vi "SplineFit.vi"(10 "Y array":dbl[](array[numeric]), 11 "X array":dbl[](array[numeric])) -> (2 "derivative":cluster{dbl[], "Best Polynomial Fit":dbl[]}[](graph), 3 "Spline":cluster{dbl[], "dX/dt":dbl[]}(graph), 4 "w_r":dbl, 5 "Point":cluster{dbl[], dbl[]})   [LabVIEW 2022 SP3]
uses:
  <vilib>/gmath/NI_Gmath.lvlib
  <vilib>/Analysis/NI_AALPro.lvlib
panel:
  out "error":i32
  out "Polynomial Coefficients":dbl[](array[numeric])
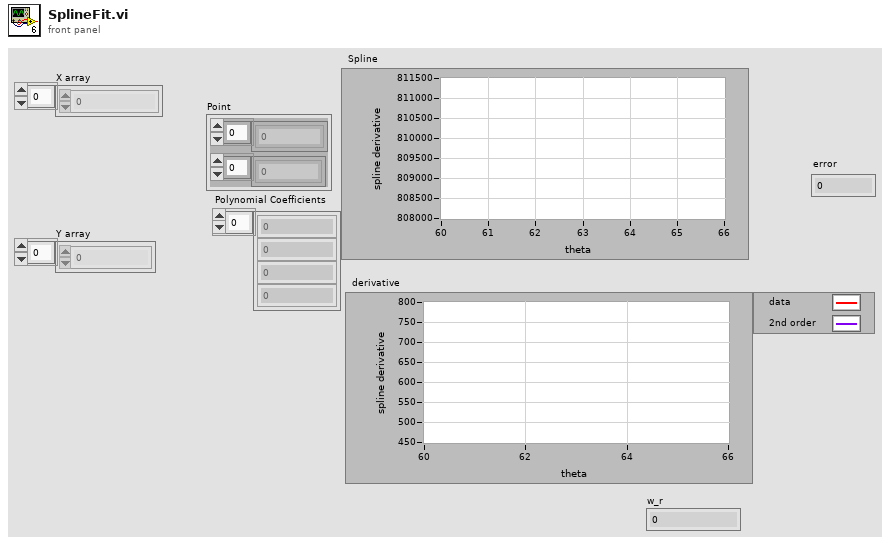
[diagram p1: front panel]
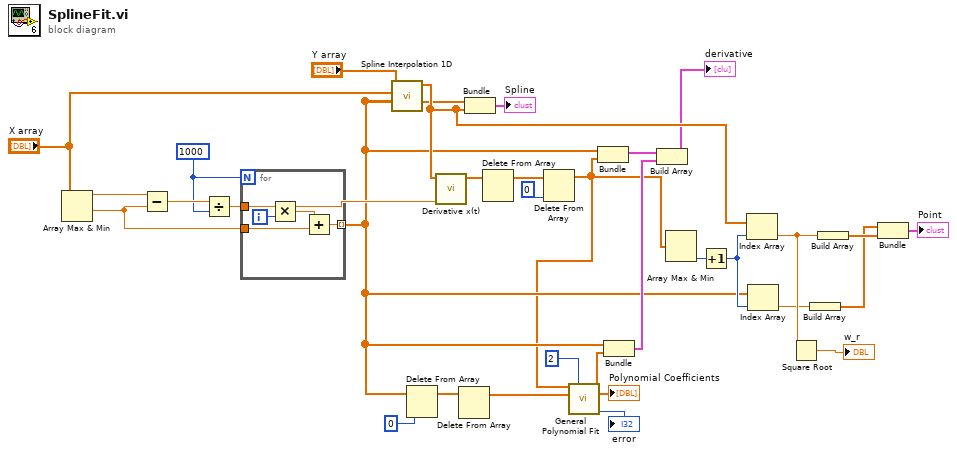
[diagram p0: block diagram]
diagram:
  w24 = 1000
  n1 = Array Max & Min(array="X array") -> (max value=w26:dbl, min value=w27:dbl)  [unwired: 2 out]
  n2 = Subtract(x=w26, y=w27) -> (x-y=w25:dbl)
  n3 = Divide(x=w25, y=w24) -> (x/y=w28:dbl)
  n4 = for {
    N: w24 -> [_]
    tunnel: w27 -> [w35]
    tunnel: w28 -> [w37]
    tunnel: [w33] -> w6 mode=indexing
    i -> [w36]
    n5 = Multiply(x=w37, y=w36) -> (x*y=w34:dbl)
    n6 = Add(x=w34, y=w35) -> (x+y=w33:dbl)
  }
  n7 = call <vilib>:"Spline Interpolation 1D.vi"("xi"=w6, "X"="X array", "Y"="Y array") -> ("yi"=w30:dbl[])  [unwired: 6 in, 2 out]
  n8 = Delete From Array(array=w6, index=0) -> (array with subset deleted=w2:dbl[])  [unwired: 1 in, 1 out]
  n9 = call <vilib>:"Derivative x(t).vi"("dt"=w28, "X"=w30) -> ("dX/dt"=w16:dbl[])  [unwired: 8 in, 1 out]
  n10 = Delete From Array(array=w2) -> (array with subset deleted=w1:dbl[])  [unwired: 2 in, 1 out]
  n11 = Bundle(w6, "yi"=w30) -> (→"Spline":cluster{dbl[], "yi":dbl[]})  [unwired: 1 in]
  n12 = Delete From Array(array=w16) -> (array with subset deleted=w17:dbl[])  [unwired: 2 in, 1 out]
  n13 = Delete From Array(array=w17, index=0) -> (array with subset deleted=w5:dbl[])  [unwired: 1 in, 1 out]
  n14 = call <vilib>:"General Polynomial Fit.vi"("Y"=w5, "polynomial order"=2, "X"=w1) -> ("Best Polynomial Fit"=w12:dbl[], "Polynomial Coefficients"=→"Polynomial Coefficients":dbl[], "error"=→"error":i32)  [unwired: 9 in, 1 out]
  n15 = Bundle(w6, "dX/dt"=w5) -> (w10:cluster{dbl[], "dX/dt":dbl[]})  [unwired: 1 in]
  n16 = Bundle(w6, "Best Polynomial Fit"=w12) -> (w9:cluster{dbl[], "Best Polynomial Fit":dbl[]})  [unwired: 1 in]
  n17 = Build Array(w10, w9) -> (→"derivative":cluster{dbl[], "Best Polynomial Fit":dbl[]}[])
  n18 = Array Max & Min(array=w5) -> (min index (indices)=w18:i32)  [unwired: 3 out]
  n19 = Increment(x=w18) -> (x+1=w19:i32)
  n20 = Index Array(array=w30, index=w19) -> (element=w31:dbl)
  n21 = Index Array(array=w6, index=w19) -> (element=w22:dbl)
  n22 = Square Root(x=w31) -> (sqrt(x)=→"w_r":dbl)
  n23 = Build Array(w22) -> (w20:dbl[])
  n24 = Build Array(w31) -> (w21:dbl[])
  n25 = Bundle(w20, w21) -> (→"Point":cluster{dbl[], dbl[]})  [unwired: 1 in]
